vi "Update.vi"(8 "error in (no error)":errorcluster, 11 "Menu in":refnum<class "Menu.lvclass">) -> (0 "error out":errorcluster, 3 "Menu out":refnum<class "Menu.lvclass">)   [LabVIEW 2019, in "RT_Game.lvlib" / "Menu.lvclass"]
uses:
  Menu.lvclass
  Game/Game.lvclass
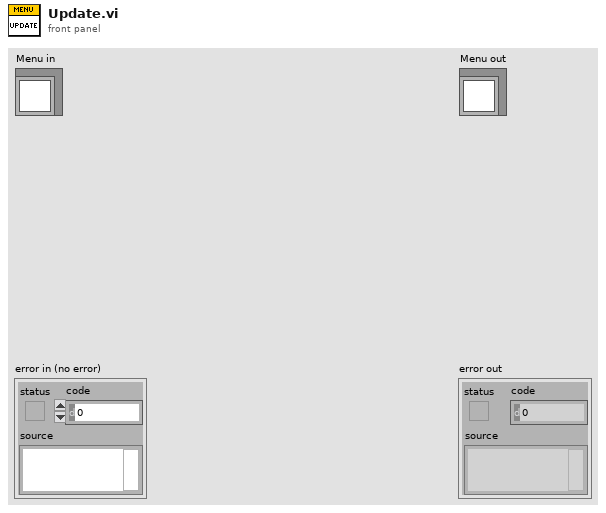
[diagram p1: front panel]
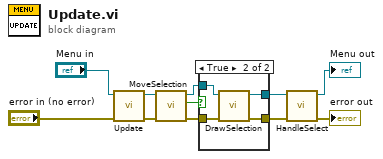
[diagram p0: block diagram]
diagram:
  n1 = call-parent "Update.vi"("error in (no error)"="error in (no error)", "Game in"="Menu in") -> ("error out"=w11:errorcluster, "Game out"=w7:refnum<class "Menu.lvclass">)  [unwired: 8 in]
  n2 = call "MoveSelection.vi"("error in (no error)"=w11, "Menu in"=w7) -> ("error out"=w8:errorcluster, "Changed?"=w1:bool, "Menu out"=w5:refnum<class "Menu.lvclass">)  [unwired: 7 in]
  n3 = case shown="True" w1 {
    tunnel: w8 -> [w12 w17]
    tunnel: [w12 w16] -> w6
    tunnel: w5 -> [w13 w15]
    tunnel: [w13 w14] -> w3
    frame False {
    }
    frame True {
      n4 = call "DrawSelection.vi"("error in (no error)"=w17, "Menu in"=w15) -> ("error out"=w16:errorcluster, "Menu out"=w14:refnum<class "Menu.lvclass">)  [unwired: 8 in]
    }
  }
  n5 = call "HandleSelect.vi"("error in (no error)"=w6, "Menu in"=w3) -> ("error out"=→"error out":errorcluster, "Menu out"=→"Menu out":refnum<class "Menu.lvclass">)  [unwired: 8 in]
